vi "Wait for Broadcast.vi"(8 "error in (no error)":errorcluster, 9 "timeout in ms (-1)":i32=-1, 11 "Broadcast Message Receiver In":refnum<class "Broadcast Message Receiver.lvclass">) -> (0 "error out":errorcluster, 1 "Timed Out?":bool, 2 "Debug Data out":refnum<class "Debug Data.lvclass">, 3 "Broadcast Message Receiver Out":refnum<class "Broadcast Message Receiver.lvclass">)   [LabVIEW 2020, in "Broadcast Message Receiver.lvclass"]
uses:
  Broadcast Message Receiver.lvclass
  Debug Data/Debug Data.lvclass
  Broadcast Message Receiver.lvclass/Broadcast Message Receiver.ctl
  Debug Data/Raw Debug Data.ctl
  Debug Data/Debug Data.lvclass/Debug Data.ctl
  <vilib>/AdvancedString/Delimited String to 1D String Array.vi
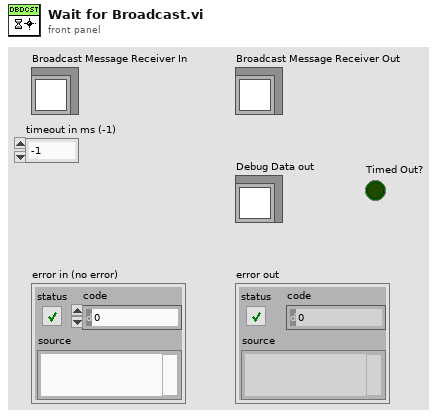
[diagram p1: front panel]
types:
  T1 = typedef "Debug Data.lvclass/Raw Debug Data.ctl" = cluster{"Action":string, "Call Chain":string, "Process":string, "Message":string, "Message Data":variant, "Time":dbl}
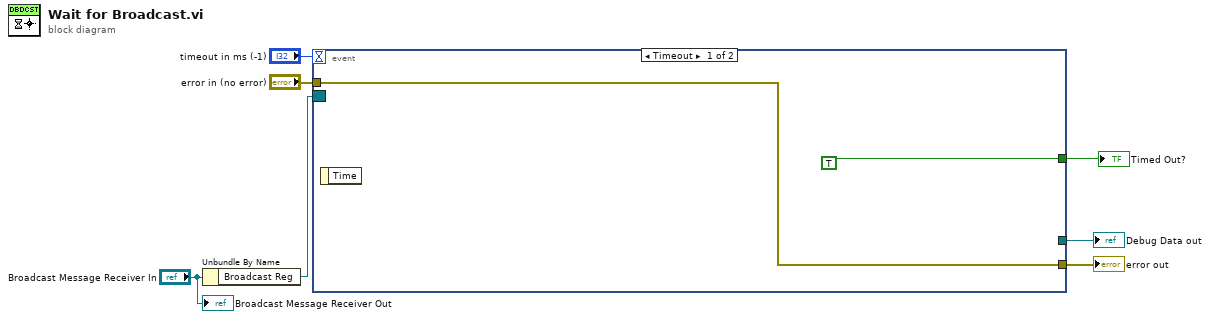
[diagram p0: block diagram]
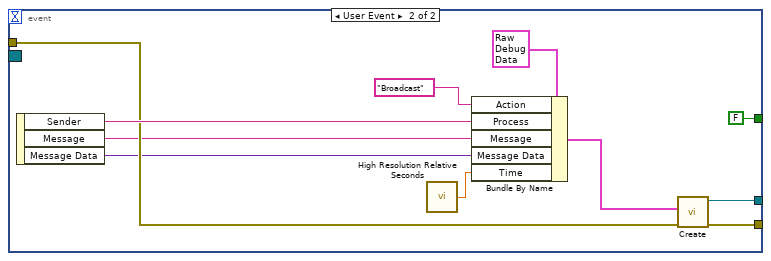
[diagram p2: hidden frame]
diagram:
  n1 = Unbundle By Name("Broadcast Message Receiver In") -> ("Broadcast Reg"=w5:refnum<event-registration>)
  n2 = event shown="[0] Timeout" {
    selector: w5 -> [_ _]
    dyn-events: _ -> [_ _]
    timeout: "timeout in ms (-1)" -> [_ _]
    tunnel: "error in (no error)" -> [w9 w12]
    tunnel: [w9 w20] -> w6
    tunnel: [_ w19] -> w7
    tunnel: [TRUE FALSE] -> w1
    event Timeout {
      n3 = event-data() -> ()  [unwired: 1 in, 1 out]
    }
    event User Event {
      n4 = event-data() -> ("Sender"=w15:string, "Message"=w10:string, "Message Data"=w11:variant)  [unwired: 1 in]
      n5 = call <vilib>:"High Resolution Relative Seconds.vi"() -> ("relative seconds"=w14:dbl)
      n6 = Bundle By Name(cluster=T1 {"Action"="", "Call Chain"="", "Process"="", "Message"="", "Message Data"=variant, "Time"=0.0} ("Debug Data Cluster"), "Action"="Broadcast", "Process"=w15, "Message"=w10, "Message Data"=w11, "Time"=w14) -> (w17:T1)
      n7 = call "Create.vi"("error in (no error)"=w12, "Debug Data Cluster"=w17) -> ("error out"=w20:errorcluster, "Debug Data out"=w19:refnum<class "Debug Data.lvclass">)  [unwired: 8 in]
    }
  }
  "Debug Data out" <- w7
  "error out" <- w6
  "Timed Out?" <- w1
  "Broadcast Message Receiver Out" <- "Broadcast Message Receiver In"
